vi "SubVI_SVM_Gaussian_Kernel.vi"(10 "sigma":dbl, 11 "X":dbl[][](array[numeric])) -> (3 "K":dbl[][](array[numeric]))   [LabVIEW 2020]
uses:
  <vilib>/Analysis/baseanly.llb/Real A x B.vi
  <vilib>/Analysis/Matrix/Numeric/Conversions/Matrix To Array - RM.vi
  <vilib>/Analysis/Matrix/Numeric/Subtract/Subtract - RM,RM.vi
  <vilib>/Analysis/Matrix/Numeric/Add/Add - RM,RM.vi
  <vilib>/Analysis/NI_AALBase.lvlib
  <vilib>/Analysis/Matrix/NI_Matrix.lvlib
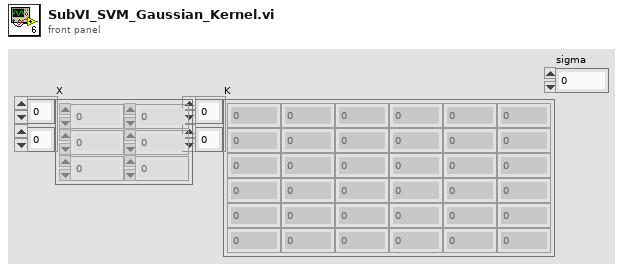
[diagram p1: front panel]
types:
  T1 = typedef "NI_Matrix.lvlib/RealMatrix.ctl" = dbl[][]
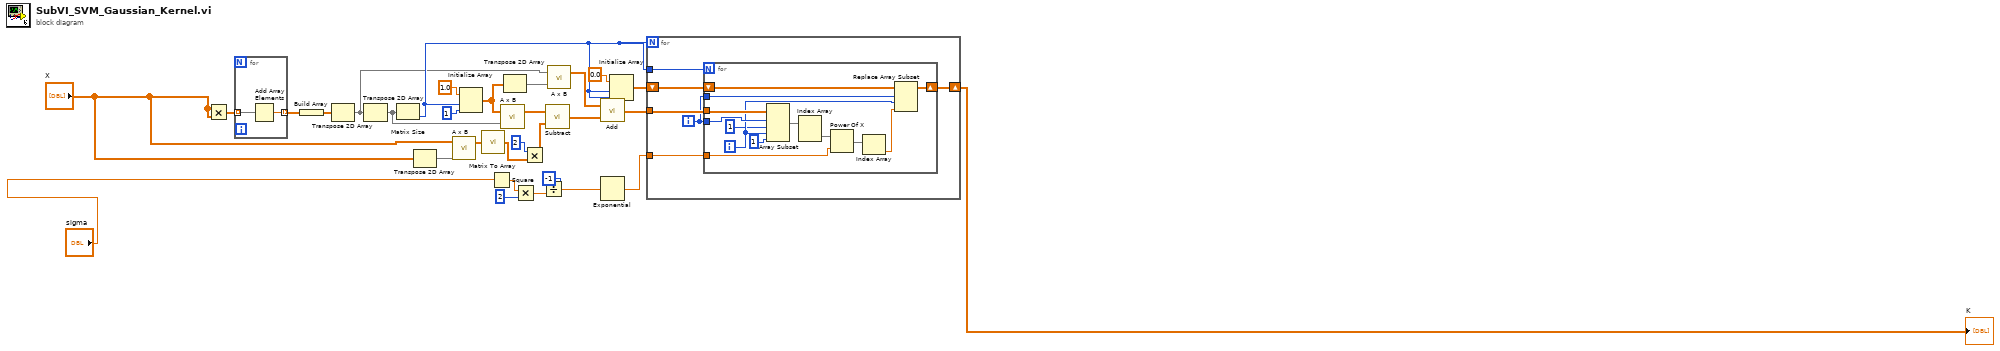
[diagram p0: block diagram]
diagram:
  n1 = Multiply(x="X", y="X") -> (x*y=w4:dbl[][])
  n2 = for {
    tunnel: w4 -> [w32] mode=indexing
    tunnel: [w31] -> w5 mode=indexing
    n3 = Add Array Elements(numeric array=w32) -> (sum=w31:dbl)
  }
  n4 = Build Array(w5) -> (w6:dbl[][])
  n5 = Transpose 2D Array(2D array=w6) -> (transposed array=w15:dbl[][])
  n6 = Transpose 2D Array(2D array=w15) -> (transposed array=w11:dbl[][])
  n7 = Matrix Size(0:w11) -> (2:w29:i32)  [unwired: 1 out]
  n8 = Transpose 2D Array(2D array="X") -> (transposed array=w7:dbl[][])
  n9 = call-poly <vilib>:"A x B.vi"("B"=w7, "A"="X") -> ("A x B"=w8:T1)  [unwired: 1 out]
  n10 = Initialize Array(1.0 ("element"), w29, 1 ("dimension size")) -> (w16:dbl[][])
  n11 = call-poly <vilib>:"Matrix To Array.vi"("Real Matrix"=w8) -> ("Real 2D Array"=w3:dbl[][])
  n12 = Square(x="sigma") -> (x^2=w20:dbl)
  n13 = call-poly <vilib>:"A x B.vi"("B"=w11, "A"=w16) -> ("A x B"=w13:T1)  [unwired: 1 out]
  n14 = Transpose 2D Array(2D array=w16) -> (transposed array=w18:dbl[][])
  n15 = Multiply(x=w20, y=2) -> (x*y=w23:dbl)
  n16 = Multiply ("Multiply.vi")(x=2 ("y"), y=w3) -> (x*y=w12:dbl[][])
  n17 = Divide(x=-1, y=w23) -> (x/y=w24:dbl)
  n18 = call-poly <vilib>:"Subtract.vi"("Real Matrix B"=w12, "Real Matrix A"=w13) -> ("A - B"=w14:T1)
  n19 = call-poly <vilib>:"A x B.vi"("B"=w18, "A"=w15) -> ("A x B"=w17:T1)  [unwired: 1 out]
  n20 = call-poly <vilib>:"Add.vi"("Real Matrix B"=w14, "Real Matrix A"=w17) -> ("A + B"=w26:T1)
  n21 = Exponential(1:w24) -> (0:w25:dbl)
  n22 = Initialize Array(0.0 ("element"), w29, w29) -> (w28:dbl[][])
  n23 = for {
    N: w29 -> [_]
    tunnel: w25 -> [w34]
    tunnel: w26 -> [w36]
    tunnel: w29 -> [w38]
    shift-right: [w33] -> w30
    shift-left: w28 -> [w37]
    i -> [w35]
    n24 = for {
      N: w38 -> [_]
      tunnel: w35 -> [w50]
      tunnel: w36 -> [w49]
      tunnel: w35 -> [w48]
      tunnel: w34 -> [w44]
      shift-right: [w45] -> w33
      shift-left: w37 -> [w51]
      i -> [w43]
      n25 = Array Subset(array=w49, index (row)=w48, length (row)=1 ("length"), index (col)=w43, length (col)=1 ("length")) -> (w40:T1)
      n26 = Index Array(array=w40) -> (element=w39:dbl[])  [unwired: 2 in]
      n27 = Power Of X(1:w44, 2:w39) -> (0:w47:dbl[])
      n28 = Index Array(array=w47) -> (element=w46:dbl)  [unwired: 1 in]
      n29 = Replace Array Subset(array=w51, new element=w46, index (row)=w50, index (col)=w43) -> (w45:dbl[][])
    }
  }
  "K" <- w30
